vi "Add string to test comments.vi"(7 "Last section (n)?":bool, 8 "error in (no error)":errorcluster, 9 "New Section (y)?":bool=TRUE, 10 "Start new response section (n)?":bool, 11 "Comments":string) -> (0 "error out":errorcluster, 3 "concatenated string":string)   [LabVIEW 2024]
uses:
  Global 2.vi
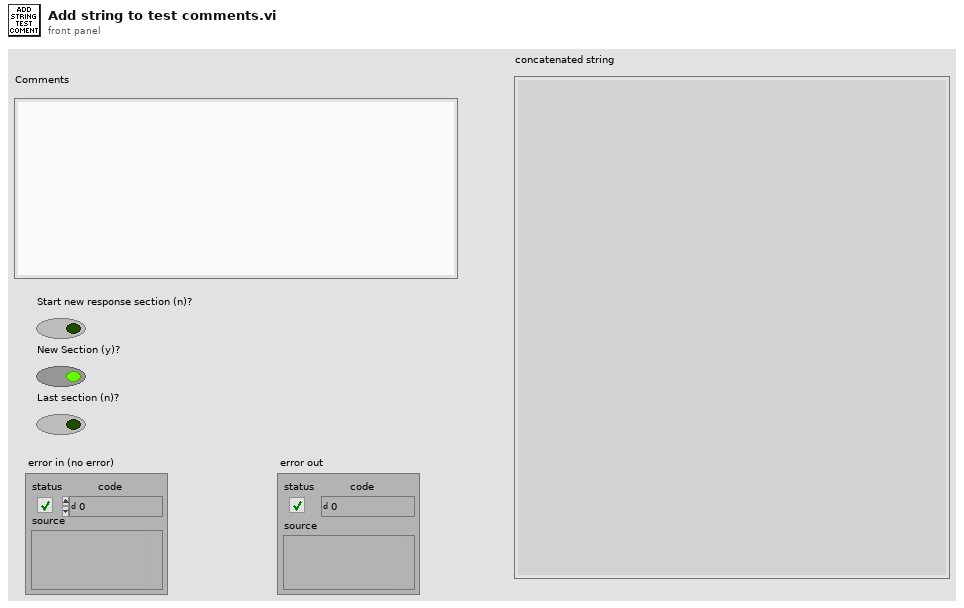
[diagram p1: front panel]
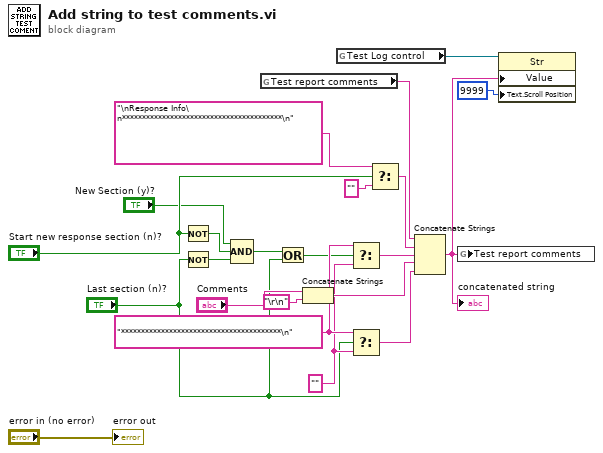
[diagram p0: block diagram]
diagram:
  w12 = "" ("f")
  w21 = "****************************************\n"
  n1 = Not(x="Start new response section (n)?") -> (.not. x?=w8:bool)
  n2 = Not(x="Last section (n)?") -> (.not. x?=w6:bool)
  n3 = Compound Arithmetic op=AND("New Section (y)?", w8, w6) -> (w5:bool)
  n4 = global read "Global 2.vi" "Test report comments"() -> (w3:string)
  n5 = Or(x=w5, y="Last section (n)?") -> (x .or. y?=w11:bool)
  n6 = Concatenate Strings("Comments", "\r\n") -> (w13:string)
  n7 = global read "Global 2.vi" "Test Log control"() -> (w4:refnum<vi>)
  n8 = Select(t=w21, s=w11, f=w12) -> (s? t:f=w16:string)
  n9 = Select(t=w21, s="Last section (n)?", f=w12) -> (s? t:f=w20:string)
  n10 = Select(t="\nResponse Info\n****************************************\n", s="Start new response section (n)?", f="") -> (s? t:f=w17:string)
  n11 = Concatenate Strings(w3, w17, w16, w13, w20) -> (w2:string)
  "concatenated string" <- w2
  n12 = global write "Global 2.vi" "Test report comments"(w2) -> ()
  n13 = property class="Str"(reference=w4, "Value"=w2, "Text.Scroll Position"=u32 9999) -> ()  [unwired: 1 in, 2 out]
  "error out" <- "error in (no error)"
